vi "Test Set Row Values Bool.vi"(11 "Test Case In":refnum<class "Test Open Xml.lvclass">) -> (0 "error out":errorcluster, 3 "Test Case Out":refnum<class "Test Open Xml.lvclass">)   [LabVIEW 2020, in "Test Open Xml.lvclass"]
uses:
  Test Open Xml.lvclass
  <vilib>/Astemes/LUnit/Test Case.lvclass
  Source/Open Xml.lvlib
  Source/Cell DataType.ctl
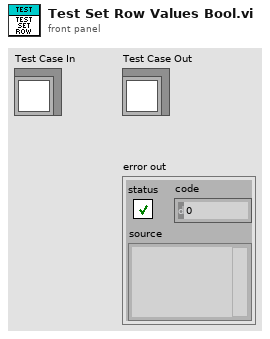
[diagram p1: front panel]
types:
  T1 = typedef "Open Xml.lvlib/Cell DataType.ctl" = enum16{"Void", "Boolean", "Number", "Error", "SharedString", "String", "InlineString", "Date"}
  T2 = cluster{"Number":dbl, "String":string, "Boolean":bool, "Time Stamp":timestamp, "Error":errorcluster}[][]
  T3 = cluster{"Number":dbl, "String":string, "Boolean":bool, "Time Stamp":timestamp, "Error":errorcluster}
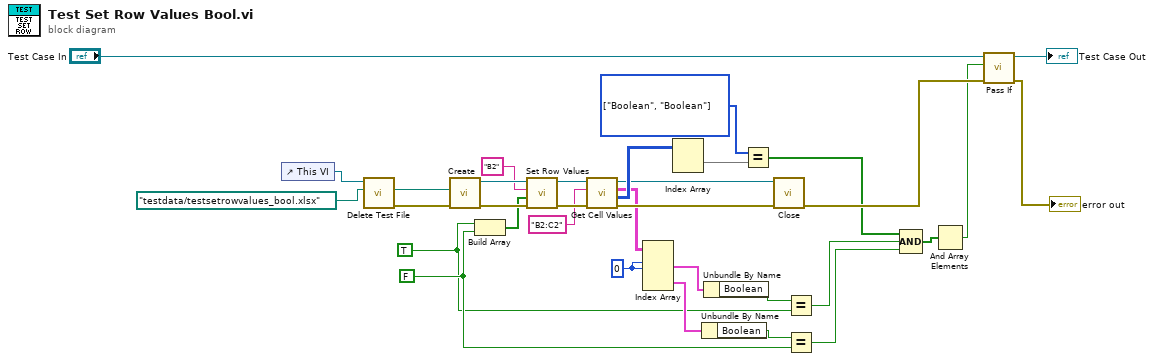
[diagram p0: block diagram]
diagram:
  w6 = 0 ("index (col)")
  w8 = TRUE
  w9 = FALSE
  w18 = T1[] [enum."Boolean", enum."Boolean"] items=["Void", "Boolean", "Number", "Error", "SharedString", "String", "InlineString", "Date"] ("x")
  n1 = control-ref of="This VI"() -> (w3:refnum<vi>)
  n2 = call "Delete Test File.vi"("name or relative path"=path "testdata/testsetrowvalues_bool.xlsx", "VI in"=w3) -> ("error out"=w4:errorcluster, "deleted path"=w1:path)  [unwired: 8 in]
  n3 = call "Create.vi"("error in"=w4, "Path"=w1) -> ("error out"=w29:errorcluster, "SpreadsheetDoc"=w30:refnum<k24>)  [unwired: 8 in]
  n4 = Build Array(w8, w9) -> (w14:bool[])
  n5 = call "Set Row Values.vi"("error in"=w29, "Values"=w14, "Cell Address"="B2", "SpreadsheetDoc"=w30) -> ("error out"=w25:errorcluster, "SpreadsheetDoc out"=w24:refnum<k24>)  [unwired: 6 in]
  n6 = call "Get Cell Values.vi"("error in"=w25, "Cell Addresses"="B2:C2" ("Cell Address"), "SpreadsheetDoc in"=w24) -> ("error out"=w27:errorcluster, "Types"=w23:T1[][], "Cell Values"=w19:T2, "SpreadsheetDoc out"=w10:refnum<k24>)  [unwired: 5 in]
  n7 = Index Array(array=w19, index (row) #1=w6, index (col) #1=w6) -> (element #1=w5:T3, element #2=w17:T3)  [unwired: 2 in]
  n8 = Index Array(array=w23) -> (element=w7:T1[])  [unwired: 2 in]
  n9 = Unbundle By Name(w17) -> ("Boolean"=w12:bool)
  n10 = Unbundle By Name(w5) -> ("Boolean"=w15:bool)
  n11 = Equal?(x=w18, y=w7) -> (x = y?=w22:bool[])
  n12 = call "Close.vi"("error in"=w27, "SpreadsheetDoc"=w10) -> ("error out"=w28:errorcluster)  [unwired: 9 in]
  n13 = Equal?(x=w15, y=w8) -> (x = y?=w11:bool)
  n14 = Equal?(x=w12, y=w9) -> (x = y?=w13:bool)
  n15 = Compound Arithmetic op=AND(w22, w11, w13) -> (w16:bool[])
  n16 = And Array Elements(Boolean array=w16) -> (logical AND=w26:bool)
  n17 = call <vilib>:"Pass If.vi"("error in (no error)"=w28, "Pass?"=w26, "LUnit Test Case In"="Test Case In") -> ("error out"=→"error out":errorcluster, "LUnit Test Case Out"=→"Test Case Out":refnum<class "Test Open Xml.lvclass">)  [unwired: 7 in]
